vi "Example 7 - While Loops (Part 2).vi"() -> ()   [LabVIEW 2015]
uses:
  source/Loop Terminal Type.ctl
  source/Scripting.lvlib
panel:
  in  "Loop Terminal Types":T1[](array[typedef])=[enum."Last Value", enum."Concatenating"]
  in  "Conditional Terminals?":bool=TRUE
  in  "Inputs Indexing?":bool[](array[boolean])=[FALSE, FALSE]
  in  "Shift Registers?":bool=TRUE
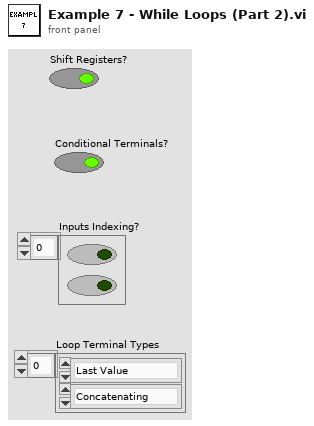
[diagram p1: front panel]
types:
  T1 = typedef "Scripting.lvlib/Loop Terminal Type.ctl" = enum16{"Last Value", "Indexing", "Concatenating"}
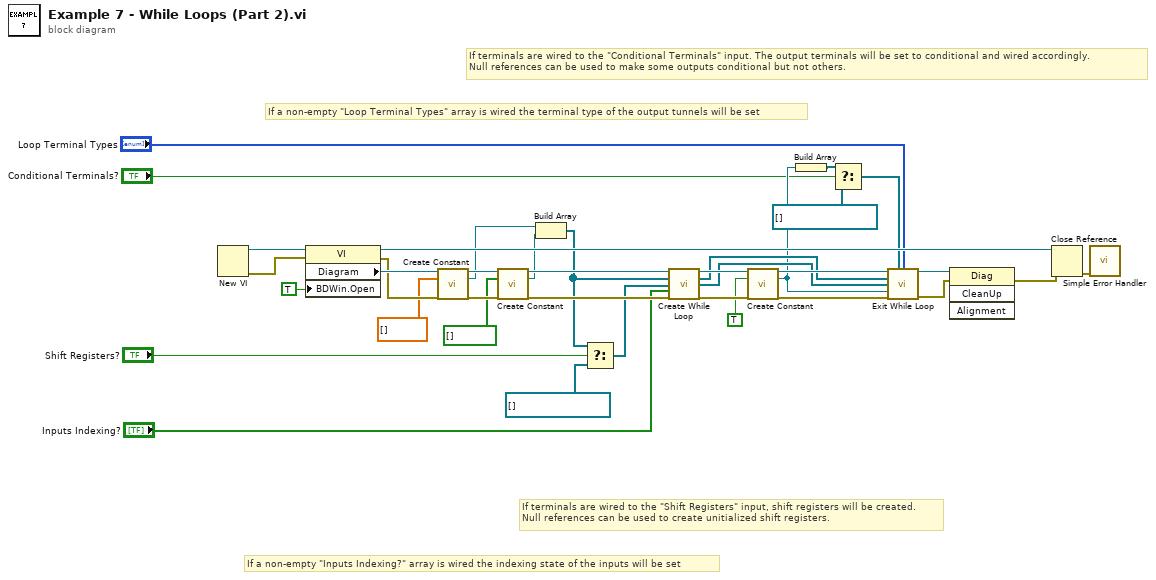
[diagram p0: block diagram]
diagram:
  # "If a non-empty \"Loop Terminal Types\" array is wired the terminal type of the output tunnels will be set"
  # "If terminals are wired to the \"Conditional Terminals\" input. The output terminals will be set to conditional and wired accordingly.\nNull references can be used to make some outputs conditional but not others."
  # "If a non-empty \"Inputs Indexing?\" array is wired the indexing state of the inputs will be set"
  # "If terminals are wired to the \"Shift Registers\" input, shift registers will be created.\nNull references can be used to create unitialized shift registers."
  n1 = New VI() -> (0:w17:errorcluster, 3:w18:refnum<vi>)  [unwired: 7 in]
  n2 = property class="VI"(reference=w18, error in=w17, "BDWin.Open"=TRUE ("Block Diagram Window:Open")) -> (reference out=w34:refnum<vi>, error out=w31:errorcluster, "Diagram"=w33:refnum<vi>)
  n3 = call "Create Constant.vi"("Diagram in"=w33, "Value"=dbl[] [], "error in (no error)"=w31) -> ("Diagram out"=w32:refnum<vi>, "Terminal"=w27:refnum<vi>, "error out"=w30:errorcluster)  [unwired: 10 in]
  n4 = call "Create Constant.vi"("Diagram in"=w32, "Value"=bool[] [], "error in (no error)"=w30) -> ("Diagram out"=w29:refnum<vi>, "Terminal"=w26:refnum<vi>, "error out"=w28:errorcluster)  [unwired: 10 in]
  n5 = Build Array(w27, w26) -> (w16:refnum<vi>[])
  n6 = Select(t=w16, s="Shift Registers?", f=refnum<vi>[] []) -> (s? t:f=w14:refnum<vi>[])
  n7 = call "Create While Loop.vi"("Diagram in"=w29, "Inputs"=w16, "Shift Register Inputs"=w14, "Inputs Indexing?"="Inputs Indexing?", "error in (no error)"=w28) -> ("Diagram out"=w25:refnum<vi>, "Inputs"=w21:refnum<vi>[], "Shift Registers"=w10:refnum<vi>[], "error out"=w24:errorcluster)  [unwired: 6 in, 1 out]
  n8 = call "Create Constant.vi"("Diagram in"=w25, "Value"=TRUE, "error in (no error)"=w24) -> ("Diagram out"=w22:refnum<vi>, "Terminal"=w6:refnum<vi>, "error out"=w20:errorcluster)  [unwired: 10 in]
  n9 = Build Array(w6) -> (w4:refnum<vi>[])
  n10 = Select(t=w4, s="Conditional Terminals?", f=refnum<vi>[] []) -> (s? t:f=w2:refnum<vi>[])
  n11 = call "Exit While Loop.vi"("Diagram in"=w22, "Conditional Terminals"=w2, "Loop Terminal Types"="Loop Terminal Types", "Outputs"=w21, "Shift Registers"=w10, "Stop Condition"=w6, "error in (no error)"=w20) -> ("Diagram out"=w12:refnum<vi>, "error out"=w11:errorcluster)  [unwired: 5 in, 2 out]
  n12 = invoke class="Diag" method="CleanUp"(reference=w12, error in=w11) -> (error out=w19:errorcluster)  [unwired: 2 in, 3 out]
  n13 = Close Reference(reference=w34, error in (no error)=w19) -> (error out=w35:errorcluster)
  n14 = call <vilib>:"Simple Error Handler.vi"("error in (no error)"=w35) -> ()  [unwired: 4 in, 5 out]
